vi "Review Result.vi"(0 "SG Path in":refnum<class "SG Abstract Path.lvclass">, 11 "error in (no error)":errorcluster) -> (4 "SG Path out":refnum<class "SG Abstract Path.lvclass">, 6 "Response":string, 15 "error out":errorcluster)   [LabVIEW 2023, in "RFFixtureCharact.Public.lvlib" / "SG Abstract Path.lvclass"]
uses:
  SG Abstract Path.lvclass
  <vilib>/Utility/error.llb/Trim Whitespace One-Sided.vi
  Scalar Path/Scalar Path.lvclass
  Common/RFCalAndFixtureCharact.Common.lvlib
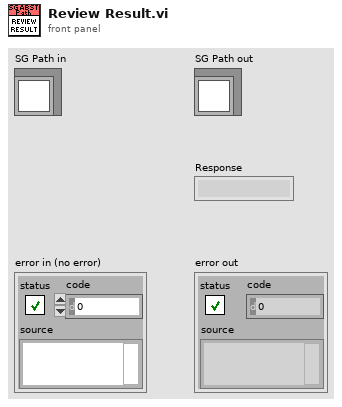
[diagram p1: front panel]
types:
  T1 = typedef "RFFixtureCharact.Public.lvlib/Scalar Path.lvclass/Scalar Charact Result.ctl" = cluster{"Port Power":dbl, "Reference Level":dbl, "Frequency":dbl, "Path Gain":dbl, "Out Of Limit":bool}
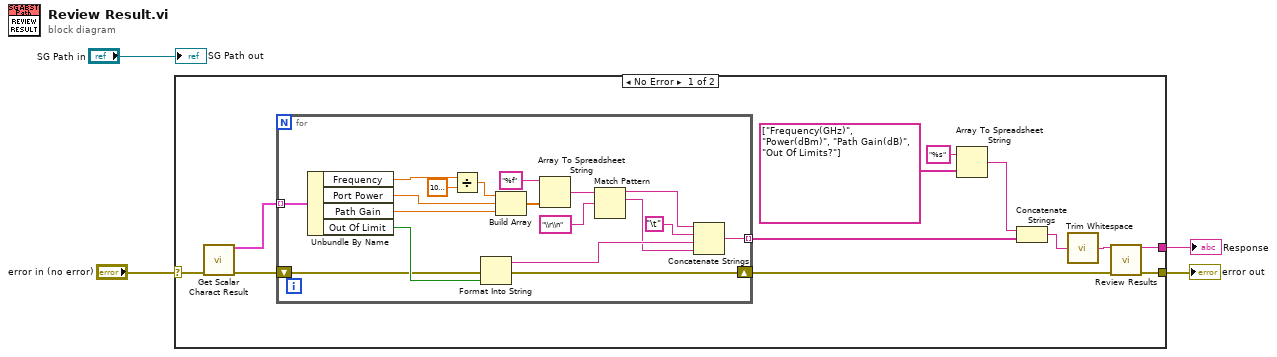
[diagram p0: block diagram]
diagram:
  n1 = case shown="No Error" "error in (no error)" {
    selector: "error in (no error)" -> [w12 w35]
    tunnel: [w13 w35] -> w3
    tunnel: [w14 _] -> w2
    frame No Error {
      n2 = call "Get Scalar Charact Result.vi"("error in (no error)"=w12) -> ("Charact result"=w16:T1[], "error out"=w11:errorcluster)  [unwired: 13 in]
      n3 = for {
        tunnel: w16 -> [w34] mode=indexing
        tunnel: [w27] -> w15 mode=indexing
        shift-right: [w22] -> w10
        shift-left: w11 -> [w23]
        n4 = Unbundle By Name(w34) -> ("Frequency"=w17:dbl, "Port Power"=w33:dbl, "Path Gain"=w32:dbl, "Out Of Limit"=w29:bool)
        n5 = Divide(x=w17, y=1000000000.0) -> (x/y=w18:dbl)
        n6 = Format Into String(error in=w23, w29) -> (resulting string=w28:string, error out=w22:errorcluster)  [unwired: 2 in]
        n7 = Build Array(w18, w33, w32) -> (w31:dbl[])
        n8 = Array To Spreadsheet String(array=w31, 3:"%f" ("format string")) -> (spreadsheet string=w25:string)  [unwired: 1 in]
        n9 = Match Pattern(string=w25, regular expression="\\r\\n") -> (before substring=w24:string, match substring=w20:string)  [unwired: 1 in, 2 out]
        n10 = Concatenate Strings(w24, "\t", w28, w20) -> (w27:string)
      }
      n11 = Array To Spreadsheet String(array=string[] ["Frequency(GHz)", "Power(dBm)", "Path Gain(dB)", "Out Of Limits?"], 3:"%s" ("format string")) -> (spreadsheet string=w5:string)  [unwired: 1 in]
      n12 = Concatenate Strings(w5, w15) -> (w9:string)
      n13 = call <vilib>:"Trim Whitespace.vi"("string"=w9) -> ("trimmed string"=w8:string)  [unwired: 1 in]
      n14 = call "Review Results.vi"("Cal Results"=w8, "error in (no error)"=w10) -> ("Response"=w14:string, "error out"=w13:errorcluster)  [unwired: 12 in]
    }
    frame Error {
    }
  }
  "error out" <- w3
  "Response" <- w2
  "SG Path out" <- "SG Path in"
